vi "Write Log File .vi"(8 "error in (no error)":errorcluster, 9 "filename":string="logfile.txt", 10 "String to Append":string, 11 "base path":path) -> (0 "error out":errorcluster)   [LabVIEW 2017]
doc: "Use this VI to add entries to a logfile such as an error log."
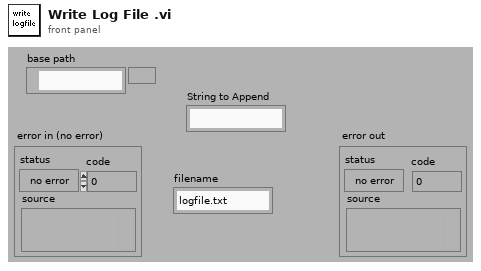
[diagram p1: front panel]
types:
  T1 = enum16{"open", "replace", "create", "open or create", "replace or create", "replace or create with confirmation"}
  T2 = typedef "Semaphore RefNum" = refnum<k1>
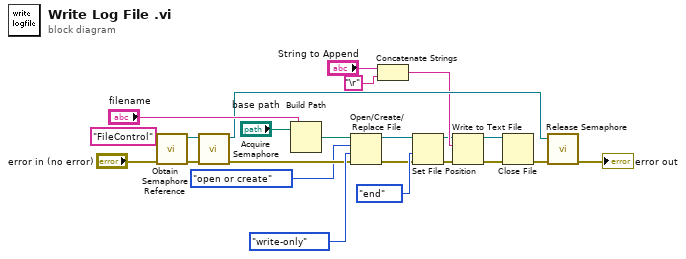
[diagram p0: block diagram]
diagram:
  n1 = call <vilib>:"Obtain Semaphore Reference.vi"("error in (no error)"="error in (no error)", "name (unnamed)"="FileControl") -> ("error out"=w15:errorcluster, "semaphore"=w14:T2)  [unwired: 1 in, 3 out]
  n2 = call <vilib>:"Acquire Semaphore.vi"("error in (no error)"=w15, "semaphore"=w14) -> ("error out"=w8:errorcluster, "semaphore out"=w11:T2)  [unwired: 1 in, 3 out]
  n3 = Build Path(base path="base path", name or relative path="filename") -> (appended path=w9:path)
  n4 = Open/Create/Replace File(file path (use dialog)=w9, error in=w8, operation (0:open)=T1."open or create", access (0:read/write)=enum16{"read/write", "read-only", "write-only"}."write-only") -> (refnum out=w4:refnum<file>, error out=w3:errorcluster)  [unwired: 3 out]
  n5 = Concatenate Strings("String to Append", "\r") -> (w5:string)
  n6 = Set File Position(refnum=w4, from (0:start)=enum16{"start", "end", "current"}."end", error in=w3) -> (refnum out=w1:refnum<file>, error out=w20:errorcluster)  [unwired: 1 out]
  n7 = Write to Text File(file (use dialog)=w1, text=w5, error in=w20) -> (refnum out=w23:refnum<file>, error out=w22:errorcluster)  [unwired: 2 out]
  n8 = Close File(refnum=w23, error in=w22) -> (error out=w16:errorcluster)  [unwired: 1 out]
  n9 = call <vilib>:"Release Semaphore.vi"("error in (no error)"=w16, "semaphore"=w11) -> ("error out"=→"error out":errorcluster)  [unwired: 5 out]
